vi "BuildPlotsOneGraph.vi"(0 "PlotCommand":string, 1 "Desired Legends":string[](array[string]), 5 "Plotstyles":T1[](array[typedef]) {"LineType" min=1 max=6 step=1; "LineWidth" min=1 max=6 step=1; "PointSize" min=0 step=0.1}, 7 "PlotNamesNeed $$?":bool=TRUE, 9 "Plot Legends":string[](array[string]), 11 "PlotArray":cluster{dbl[], dbl[]}[](array[cluster]), 12 "Legend":string[](array[string]), 13 "Error Bar Cluster":cluster{string[]}[](array[cluster])) -> (4 "String out":string, 6 "Xspan":cluster{"Max":dbl, "Min":dbl}, 10 "Yspan":cluster{"Max":dbl, "Min":dbl})   [LabVIEW 2014]
uses:
  plotstyle.ctl
  Results_plotter_Global.vi
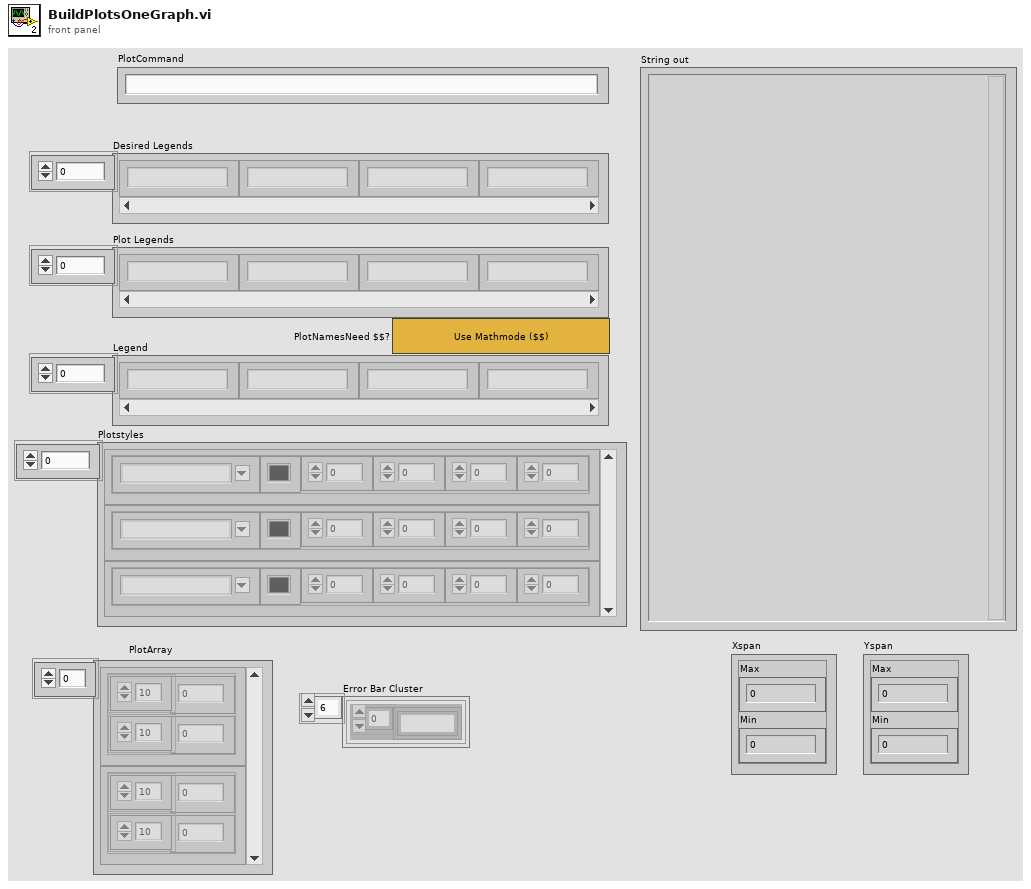
[diagram p1: front panel]
types:
  T1 = typedef "plotstyle.ctl" = cluster{"Style":string, "Color":u32, "PointType":i32, "PointSize":sgl, "LineWidth":sgl, "LineType":u8}
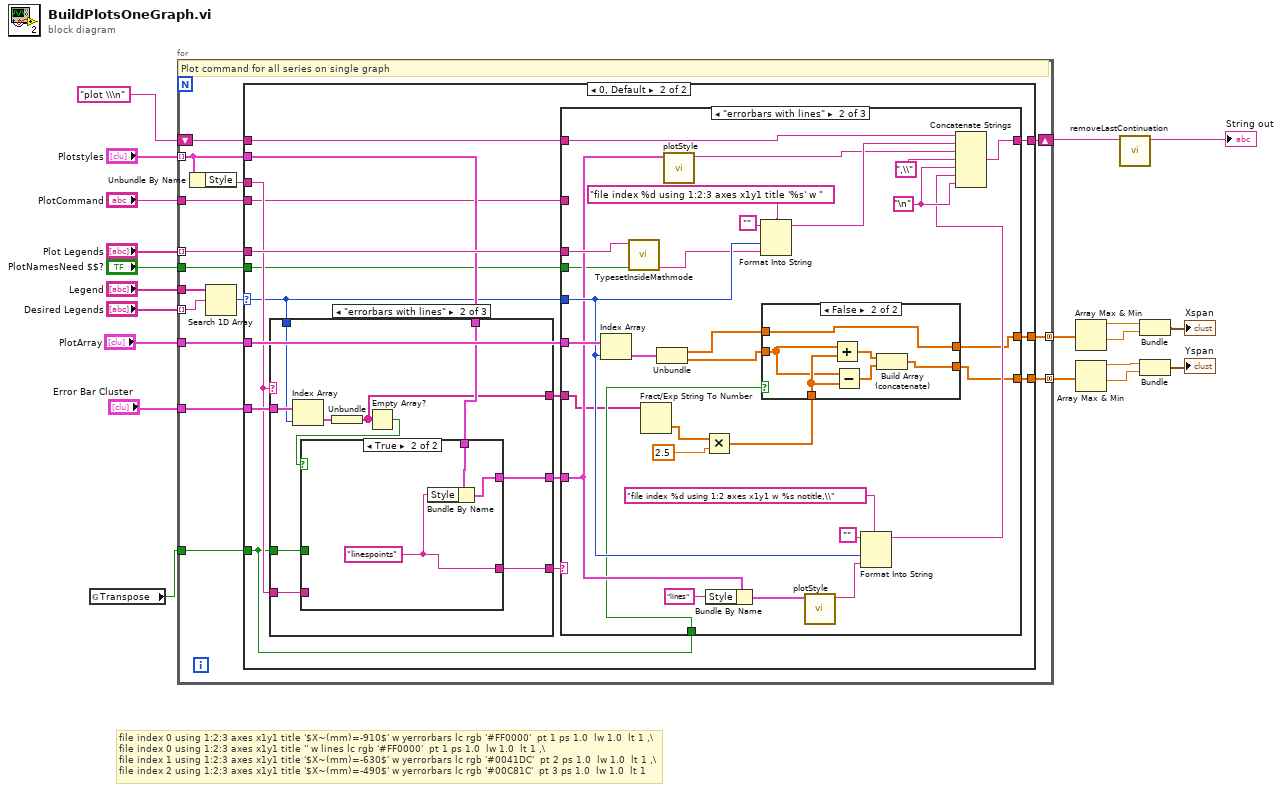
[diagram p0: block diagram]
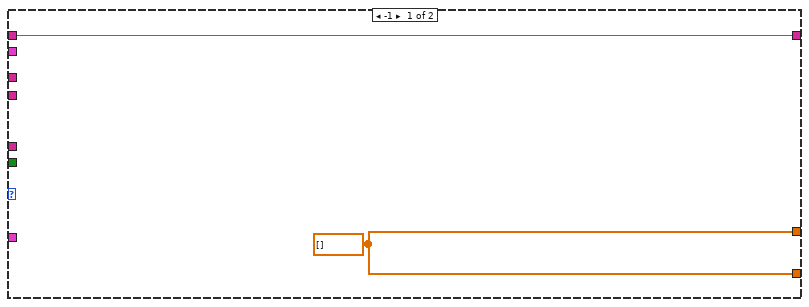
[diagram p2: hidden frame]
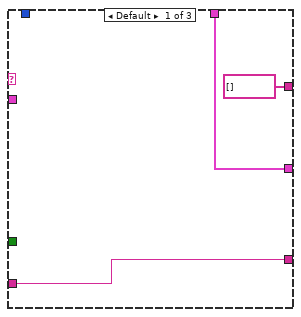
[diagram p3: hidden frame]
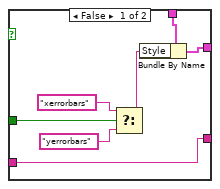
[diagram p4: hidden frame]
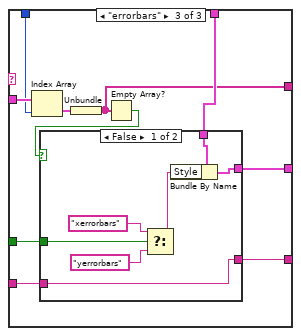
[diagram p5: hidden frame]
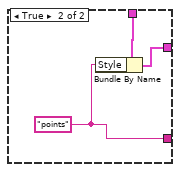
[diagram p6: hidden frame]
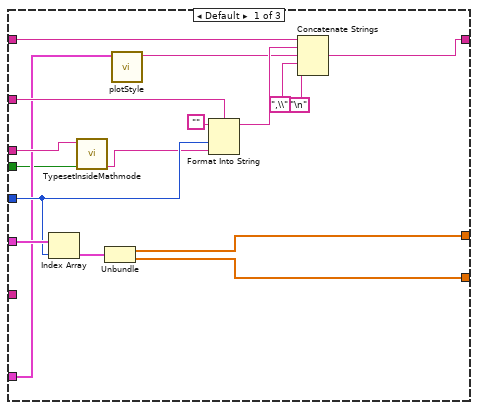
[diagram p7: hidden frame]
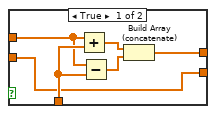
[diagram p8: hidden frame]
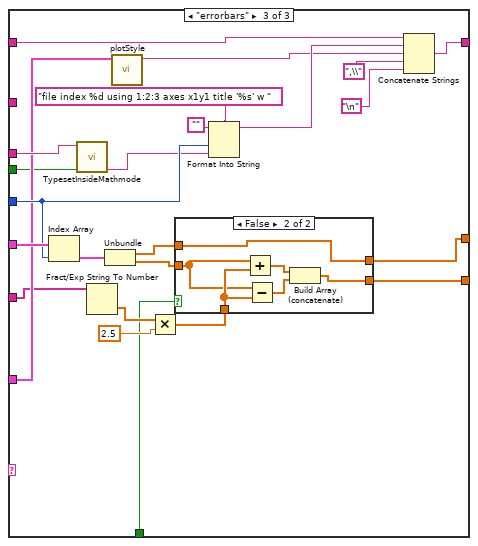
[diagram p9: hidden frame]
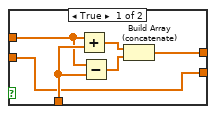
[diagram p10: hidden frame]
diagram:
  # "file index 0 using 1:2:3 axes x1y1 title '$X~(mm)=-910$' w yerrorbars lc rgb '#FF0000'  pt 1 ps 1.0  lw 1.0  lt 1 ,\\\nfile index 0 using 1:2:3 axes x1y1 title '' w lines lc rgb '#FF0000'  pt 1 ps 1.0  lw 1.0  lt 1 ,\\\nfile index 1 using 1:2:3 axes x1y1 title '$X~(mm)=-630$' w yerrorbars lc rgb '#0041DC'  pt 2 ps 1.0  lw 1.0  lt 1 ,\\\nfile index 2 using 1:2:3 axes x1y1 title '$X~(mm)=-490$' w yerrorbars lc rgb '#00C81C'  pt 3 ps 1.0  lw 1.0  lt 1"
  n1 = global read "Results_plotter_Global.vi" "Transpose"() -> (w2:bool)
  n2 = for {
    tunnel: "Plotstyles" -> [w25] mode=indexing
    tunnel: "Plot Legends" -> [w33] mode=indexing
    shift-right: [w34] -> w18
    shift-left: "plot \\\n" -> [w35]
    tunnel: "Desired Legends" -> [w31] mode=indexing
    tunnel: "Legend" -> [w32]
    tunnel: "PlotCommand" -> [w29]
    tunnel: "PlotArray" -> [w28]
    tunnel: [w27] -> w11 mode=concatenating
    tunnel: [w26] -> w10 mode=concatenating
    tunnel: "Error Bar Cluster" -> [w23]
    tunnel: w2 -> [w22]
    tunnel: "PlotNamesNeed $$?" -> [w21]
    # "Plot command for all series on single graph"
    n3 = Unbundle By Name(w25) -> ("Style"=w24:string)
    n4 = Search 1D Array(1D array=w32, element=w31) -> (index of element=w30:i32)  [unwired: 1 in]
    n5 = case shown="0, Default" w30 {
      selector: w30 -> [_ w42]
      tunnel: w25 -> [_ w46]
      tunnel: w35 -> [w37 w53]
      tunnel: [w37 w52] -> w34
      tunnel: w33 -> [_ w48]
      tunnel: w29 -> [_ w40]
      tunnel: w28 -> [_ w51]
      tunnel: [w36 w50] -> w27
      tunnel: [w36 w49] -> w26
      tunnel: w24 -> [_ w43]
      tunnel: w23 -> [_ w47]
      tunnel: w22 -> [_ w39]
      tunnel: w21 -> [_ w38]
      frame -1 {
        w36 = dbl[] []
      }
      frame 0, Default {
        n6 = case shown="\"errorbars with lines\"" w43 {
          tunnel: w47 -> [_ w66 w86]
          tunnel: w46 -> [w56 w61 w81]
          tunnel: [w56 w60 w80] -> w45
          tunnel: [w55 w63 w83] -> w44
          tunnel: w39 -> [_ w62 w82]
          tunnel: w43 -> [w55 w59 w79]
          tunnel: w42 -> [_ w58 w78]
          tunnel: [string[] [] w57 w77] -> w41
          frame Default {
          }
          frame "errorbars with lines" {
            n7 = Index Array(array=w66, index=w58) -> (element=w65:cluster{string[]})
            n8 = Unbundle(w65) -> (w57:string[])
            n9 = Empty Array?(array=w57) -> (empty?=w64:bool)
            n10 = case shown="True" w64 {
              tunnel: [w67 w74] -> w63
              tunnel: w62 -> [w71 _]
              tunnel: w61 -> [w70 w76]
              tunnel: [w69 w75] -> w60
              tunnel: w59 -> [w67 _]
              frame False {
                n11 = Select(t="xerrorbars", s=w71, f="yerrorbars") -> (s? t:f=w68:string)
                n12 = Bundle By Name(cluster=w70, "Style"=w68) -> (w69:T1)
              }
              frame True {
                w74 = "linespoints" ("Style")
                n13 = Bundle By Name(cluster=w76, "Style"=w74) -> (w75:T1)
              }
            }
          }
          frame "errorbars" {
            n14 = Index Array(array=w86, index=w78) -> (element=w85:cluster{string[]})
            n15 = Unbundle(w85) -> (w77:string[])
            n16 = Empty Array?(array=w77) -> (empty?=w84:bool)
            n17 = case shown="False" w84 {
              tunnel: [w87 w94] -> w83
              tunnel: w82 -> [w91 _]
              tunnel: w81 -> [w90 w96]
              tunnel: [w89 w95] -> w80
              tunnel: w79 -> [w87 _]
              frame False {
                n18 = Select(t="xerrorbars", s=w91, f="yerrorbars") -> (s? t:f=w88:string)
                n19 = Bundle By Name(cluster=w90, "Style"=w88) -> (w89:T1)
              }
              frame True {
                w94 = "points" ("Style")
                n20 = Bundle By Name(cluster=w96, "Style"=w94) -> (w95:T1)
              }
            }
          }
        }
        n21 = case shown="\"errorbars with lines\"" w44 {
          tunnel: w53 -> [w108 w139 w175]
          tunnel: [w99 w138 w174] -> w52
          tunnel: w40 -> [w107 _ _]
          tunnel: w51 -> [w106 w137 w173]
          tunnel: w42 -> [w105 w131 w169]
          tunnel: [w103 w117 w160] -> w50
          tunnel: [w102 w116 w159] -> w49
          tunnel: w48 -> [w101 w135 w171]
          tunnel: w45 -> [w100 w126 w167]
          tunnel: w41 -> [_ w119 w166]
          tunnel: w39 -> [_ w124 w163]
          tunnel: w38 -> [w98 w115 w157]
          frame Default {
            n22 = Index Array(array=w106, index=w105) -> (element=w104:cluster{dbl[], dbl[]})
            n23 = call "TypesetInsideMathmode.vi"("Needs $$?"=w98, "DirtyString"=w101) -> ("ChosenStringtype"=w97:string)  [unwired: 7 in, 2 out]
            n24 = Unbundle(w104) -> (w103:dbl[], w102:dbl[])
            n25 = call "plotStyle.vi"("plotSpec"=w100) -> ("String"=w110:string)  [unwired: 10 in]
            n26 = Format Into String(format string=w107, initial string="", w105, w97) -> (resulting string=w111:string)  [unwired: 1 in, 1 out]
            n27 = Concatenate Strings(w108, w111, w110, ",\\" ("string"), "\n") -> (w99:string)
          }
          frame "errorbars with lines" {
            w127 = "\n"
            n28 = Index Array(array=w137, index=w131) -> (element=w136:cluster{dbl[], dbl[]})
            n29 = call "TypesetInsideMathmode.vi"("Needs $$?"=w115, "DirtyString"=w135) -> ("ChosenStringtype"=w114:string)  [unwired: 7 in, 2 out]
            n30 = Fract/Exp String To Number(string=w119) -> (number=w121:dbl[])  [unwired: 3 in, 1 out]
            n31 = Unbundle(w136) -> (w123:dbl[], w122:dbl[])
            n32 = call "plotStyle.vi"("plotSpec"=w126) -> ("String"=w140:string)  [unwired: 10 in]
            n33 = Multiply(x=w121, y=2.5) -> (x*y=w118:dbl[])
            n34 = Bundle By Name(cluster=w126, "Style"="lines") -> (w130:T1)
            n35 = Format Into String(format string="file index %d using 1:2:3 axes x1y1 title '%s' w ", initial string="", w131, w114) -> (resulting string=w141:string)  [unwired: 1 in, 1 out]
            n36 = case shown="False" w124 {
              tunnel: w123 -> [w146 w152]
              tunnel: w118 -> [w147 w153]
              tunnel: [w145 w152] -> w117
              tunnel: [w144 w150] -> w116
              tunnel: w122 -> [w144 w151]
              frame True {
                n37 = Add(x=w146, y=w147) -> (x+y=w148:dbl[])
                n38 = Subtract(x=w146, y=w147) -> (x-y=w149:dbl[])
                n39 = Build Array (concatenate)(w148, w149) -> (w145:dbl[])
              }
              frame False {
                n40 = Add(x=w151, y=w153) -> (x+y=w154:dbl[])
                n41 = Subtract(x=w151, y=w153) -> (x-y=w155:dbl[])
                n42 = Build Array (concatenate)(w154, w155) -> (w150:dbl[])
              }
            }
            n43 = call "plotStyle.vi"("plotSpec"=w130) -> ("String"=w128:string)  [unwired: 10 in]
            n44 = Format Into String(format string="file index %d using 1:2 axes x1y1 w %s notitle,\\", initial string="", w131, w128) -> (resulting string=w125:string)  [unwired: 1 in, 1 out]
            n45 = Concatenate Strings(w139, w141, w140, ",\\" ("string"), w127, w125, w127) -> (w138:string)
          }
          frame "errorbars" {
            n46 = Index Array(array=w173, index=w169) -> (element=w172:cluster{dbl[], dbl[]})
            n47 = call "TypesetInsideMathmode.vi"("Needs $$?"=w157, "DirtyString"=w171) -> ("ChosenStringtype"=w156:string)  [unwired: 7 in, 2 out]
            n48 = Fract/Exp String To Number(string=w166) -> (number=w165:dbl[])  [unwired: 3 in, 1 out]
            n49 = Unbundle(w172) -> (w162:dbl[], w158:dbl[])
            n50 = call "plotStyle.vi"("plotSpec"=w167) -> ("String"=w176:string)  [unwired: 10 in]
            n51 = Multiply(x=w165, y=2.5) -> (x*y=w161:dbl[])
            n52 = case shown="False" w163 {
              tunnel: w162 -> [w182 w188]
              tunnel: w161 -> [w183 w189]
              tunnel: [w181 w188] -> w160
              tunnel: [w180 w186] -> w159
              tunnel: w158 -> [w180 w187]
              frame True {
                n53 = Add(x=w182, y=w183) -> (x+y=w184:dbl[])
                n54 = Subtract(x=w182, y=w183) -> (x-y=w185:dbl[])
                n55 = Build Array (concatenate)(w184, w185) -> (w181:dbl[])
              }
              frame False {
                n56 = Add(x=w187, y=w189) -> (x+y=w190:dbl[])
                n57 = Subtract(x=w187, y=w189) -> (x-y=w191:dbl[])
                n58 = Build Array (concatenate)(w190, w191) -> (w186:dbl[])
              }
            }
            n59 = Format Into String(format string="file index %d using 1:2:3 axes x1y1 title '%s' w ", initial string="", w169, w156) -> (resulting string=w177:string)  [unwired: 1 in, 1 out]
            n60 = Concatenate Strings(w175, w177, w176, ",\\" ("string"), "\n") -> (w174:string)
          }
        }
      }
    }
  }
  n61 = Array Max & Min(array=w11) -> (max value=w8:dbl, min value=w7:dbl)  [unwired: 2 out]
  n62 = Array Max & Min(array=w10) -> (max value=w6:dbl, min value=w5:dbl)  [unwired: 2 out]
  n63 = call "removeLastContinuation.vi"("String in"=w18) -> ("String out"=→"String out":string)  [unwired: 10 in]
  n64 = Bundle(w8, w7) -> (→"Xspan":cluster{dbl, dbl})  [unwired: 1 in]
  n65 = Bundle(w6, w5) -> (→"Yspan":cluster{dbl, dbl})  [unwired: 1 in]
